vi "Savitsky Golay Filter (multiple).vi"(6 "Side Points Unit (points)":enum16{"Points", "Data"}(ring), 8 "error in (no error)":errorcluster, 9 "polynomial order (3)":i32=3, 10 "side points (6)":dbl=6.0, 11 "XY-data":cluster{"X-array":dbl[], "Y-array":dbl[]}[](array[cluster])) -> (0 "error out":errorcluster, 3 "XY-data out":cluster{"X-array":dbl[], "Y-array":dbl[]}[](array[cluster]) {"Y-array" format="%.2p"; "X-array" format="%.2p"})   [LabVIEW 2019, in "xy_utilities.lvlib"]
doc: "Filter <b>XY-data</b>'s Y-Array with a Savitsky-Golay FIR smoothing filter.\n\n<b>side points</b> specifies the number of data points to each side of the current data point to use for the least squares minimization. side points*2 + 1 is the length of the moving window, which must be greater than the polynomial order.\n\n<b>polynomial order</b> specifies the order of the polynomial. \n\nWire data to the data input to determine the polymorphic instance to use or manually select the instance."
uses:
  xy_utilities.lvlib
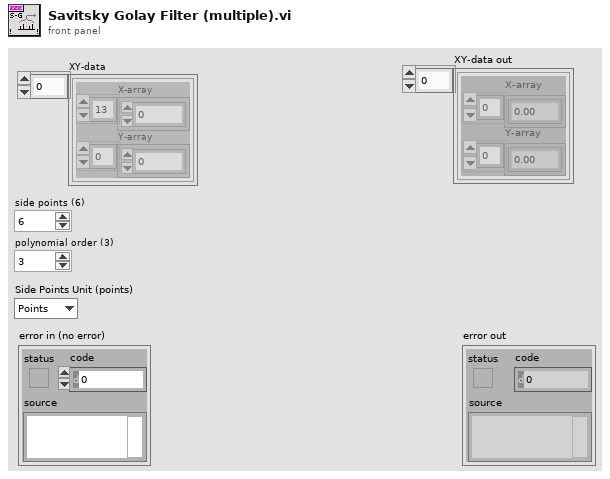
[diagram p1: front panel]
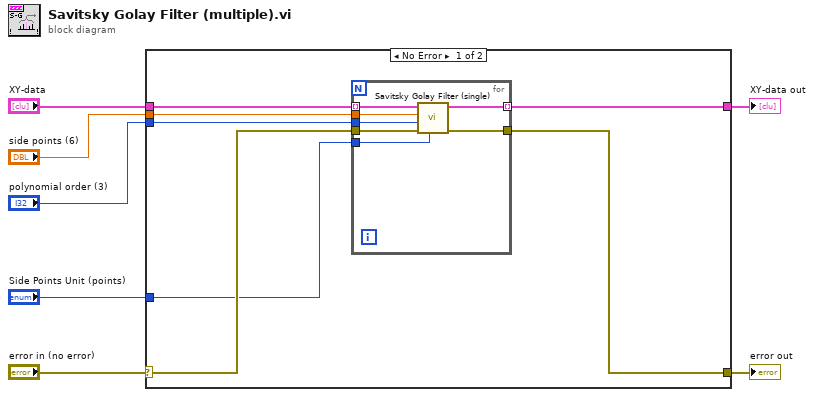
[diagram p0: block diagram]
diagram:
  n1 = case shown="No Error" "error in (no error)" {
    selector: "error in (no error)" -> [w11 w23]
    tunnel: [w10 w23] -> w6
    tunnel: "XY-data" -> [w14 w22]
    tunnel: [w13 w22] -> w4
    tunnel: "side points (6)" -> [w12 _]
    tunnel: "Side Points Unit (points)" -> [w9 _]
    tunnel: "polynomial order (3)" -> [w8 _]
    frame No Error {
      n2 = for {
        tunnel: w14 -> [w21] mode=indexing
        tunnel: [w20] -> w13 mode=indexing
        tunnel: w12 -> [w19]
        tunnel: w11 -> [w18]
        tunnel: [w17] -> w10
        tunnel: w9 -> [w16]
        tunnel: w8 -> [w15]
        n3 = call "Savitsky Golay Filter (single).vi"("Side Points Unit (points)"=w16, "error in (no error)"=w18, "polynomial order (3)"=w15, "side points (6)"=w19, "XY-data"=w21) -> ("error out"=w17:errorcluster, "XY-data out"=w20:cluster{"X-array":dbl[], "Y-array":dbl[]})  [unwired: 5 in]
      }
    }
    frame Error {
    }
  }
  "error out" <- w6
  "XY-data out" <- w4
